vi "State Logic.vi"(0 "TLB' data in":refnum<class "TLB` - {TMPL}.lvclass">, 1 "process state logic enable":bool, 5 "trigger queue in":refnum<queue>, 7 "action queue in":refnum<queue>, 11 "error in":errorcluster) -> (4 "TLB' data out":refnum<class "TLB` - {TMPL}.lvclass">, 15 "error out":errorcluster)   [LabVIEW 2016, in "TLB` Template.lvlib" / "TLB` - {TMPL}.lvclass"]
doc: "Control process for TLB' template.\n\n<B>Input Parameters</B>\n\n<B>TLB' data in</B> is the templates' private data.\n\n<B>process state logic enable</B> enable state logic change.\n\n<B>trigger queue in</B> is a reference to a queue. Use the Create Trigger Queue function to obtain a queue reference. \n\n<B>action queue in</B> is a reference to a queue. Use the Create Action Queue function to obtain a queue reference. \n\n<B>timeout (ms)</B> queue timeout.\n\n<B>error in</B> describes error conditions that occur before this node runs. This input provides standard error in functionality.\n\n<B>Output Parameters</B>\n\n<B>TLB' data out</B> is the templates' private data.\n\n<B>error out</B> contains error information. This output provides standard error out functionality."
uses:
  TLB` - {TMPL}.lvclass
  Application Components/Trigger API/System Trigger Element.ctl
  Application Components/Trigger API/{TMPL} System Trigger.ctl
  Core Components/Actions/System Action Element.ctl
  TLB` - {TMPL}.lvclass/TLB` - {TMPL}.ctl
  State.ctl
  Core Components/Error Handler/TLB` Error Handler.lvclass/TLB` Error Handler.ctl
  Core Components/Error Handler/accessors/Get Action Causing Error.vi
  Core Components/Error Handler/accessors/Get Originating State.vi
  Core Components/Error Handler/accessors/Get Destination State.vi
  Core Components/Error Handler/accessors/Get Executed System Actions.vi
  Core Components/Error Handler/accessors/Get Remaing System Actions.vi
  Core Components/Error Handler/Core/actions/support/Error FLUSH-LOG-DIALOG.vi
  Core Components/Error Handler/Core/actions/support/Error DIALOG.vi
  Application Components/Trigger API/{TMPL} Trigger API.lvlib
  Core Components/Error Handler/TLB` Error Handler.lvclass
  Core Components/Actions/Actions.lvlib
  Core Components/Error Handler/Core/actions/support/Error FLUSH-DIALOG.vi
  TLB` Template.lvlib
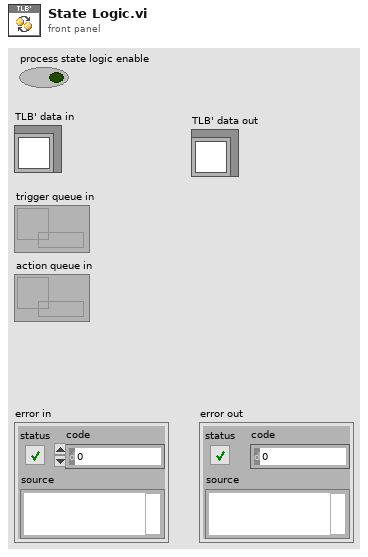
[diagram p1: front panel]
types:
  T1 = typedef "TLB` Template.lvlib/{TMPL} System Trigger.ctl" = enum16{"None", "Connect", "Start Acquisition", "Stop Acquisition", "Disconnect", "Return to Safe State Actions", "Cache User Parameters", "Close Application", "<Error>"}
  T2 = typedef "TLB` Template.lvlib/TLB` - {TMPL}.lvclass/State.ctl" = enum16{"<Startup>", "Idle", "<Shutdown>", "<Error>"}
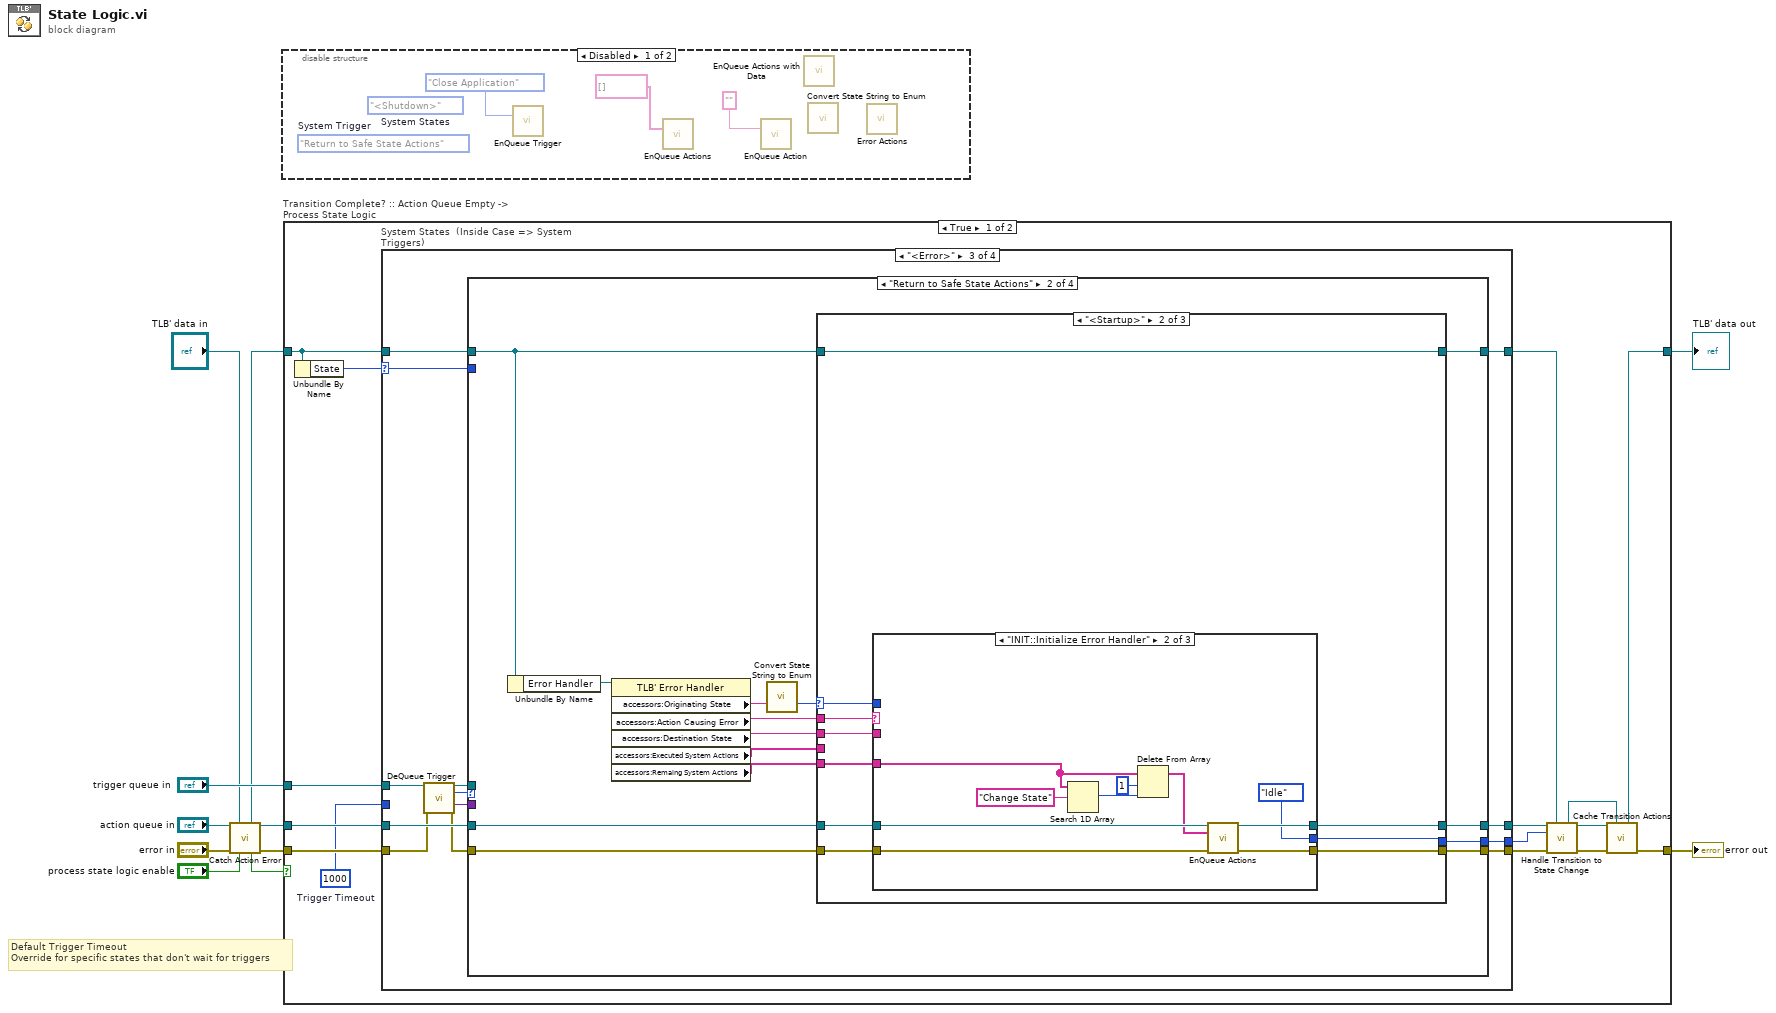
[diagram p0: block diagram]
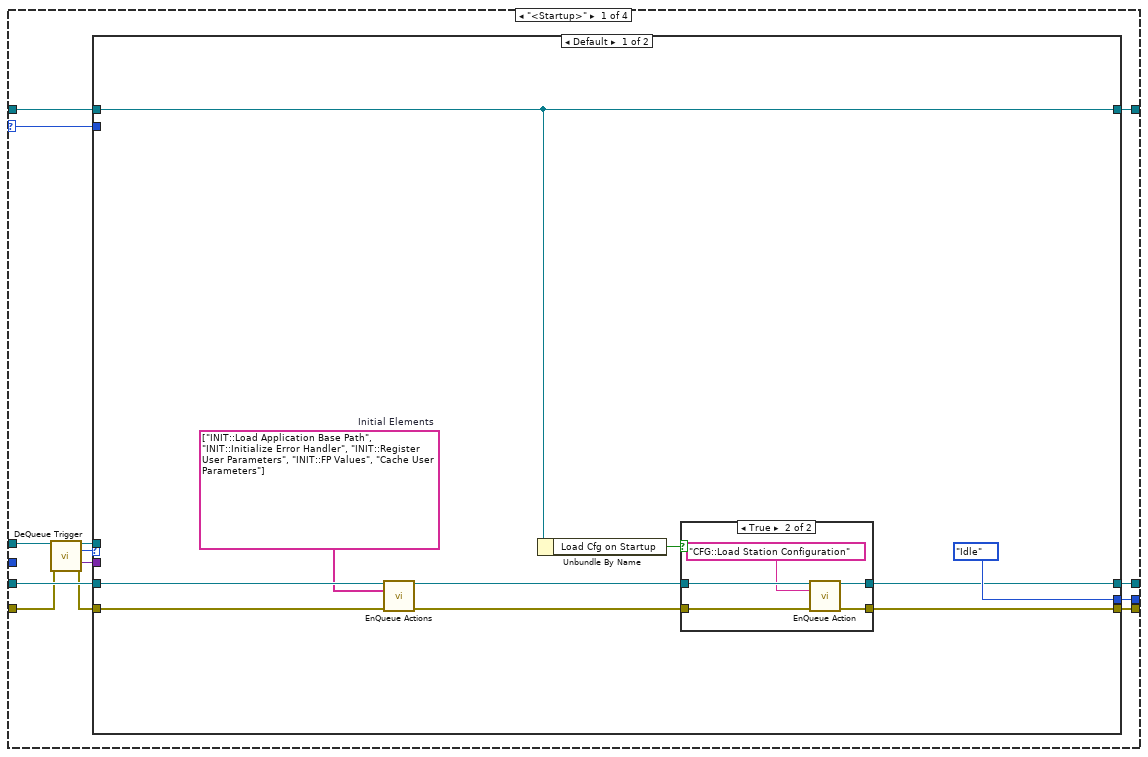
[diagram p3: hidden frame]
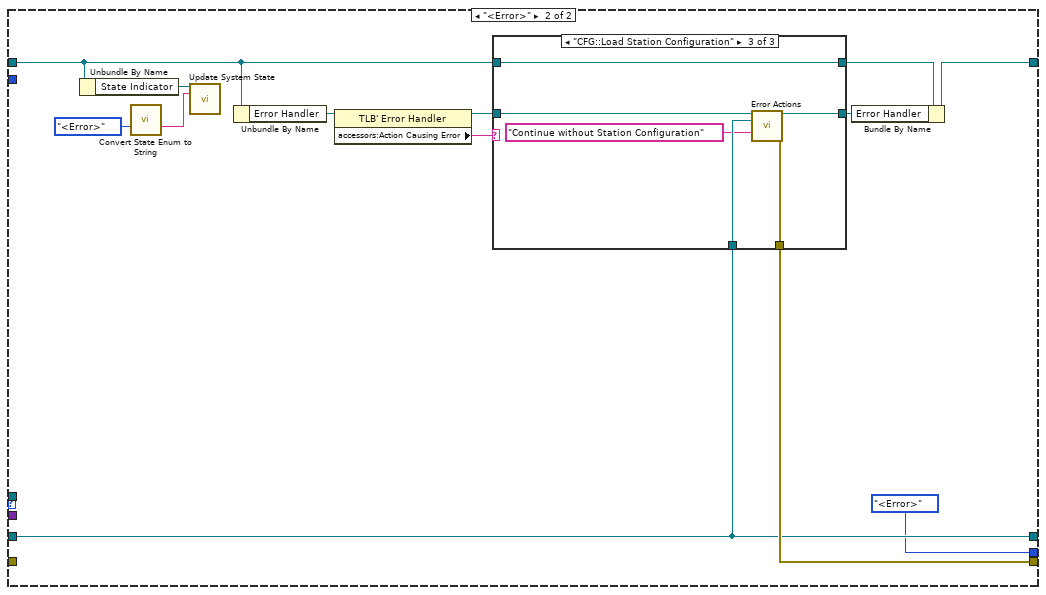
[diagram p5: hidden frame]
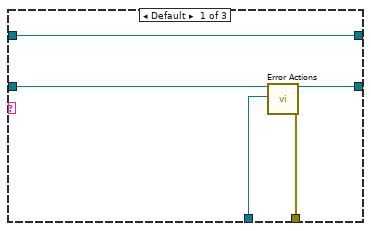
[diagram p6: hidden frame]
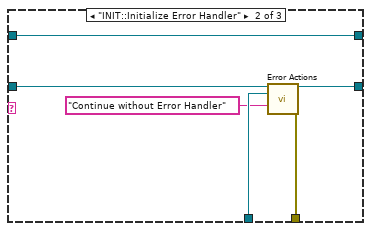
[diagram p7: hidden frame]
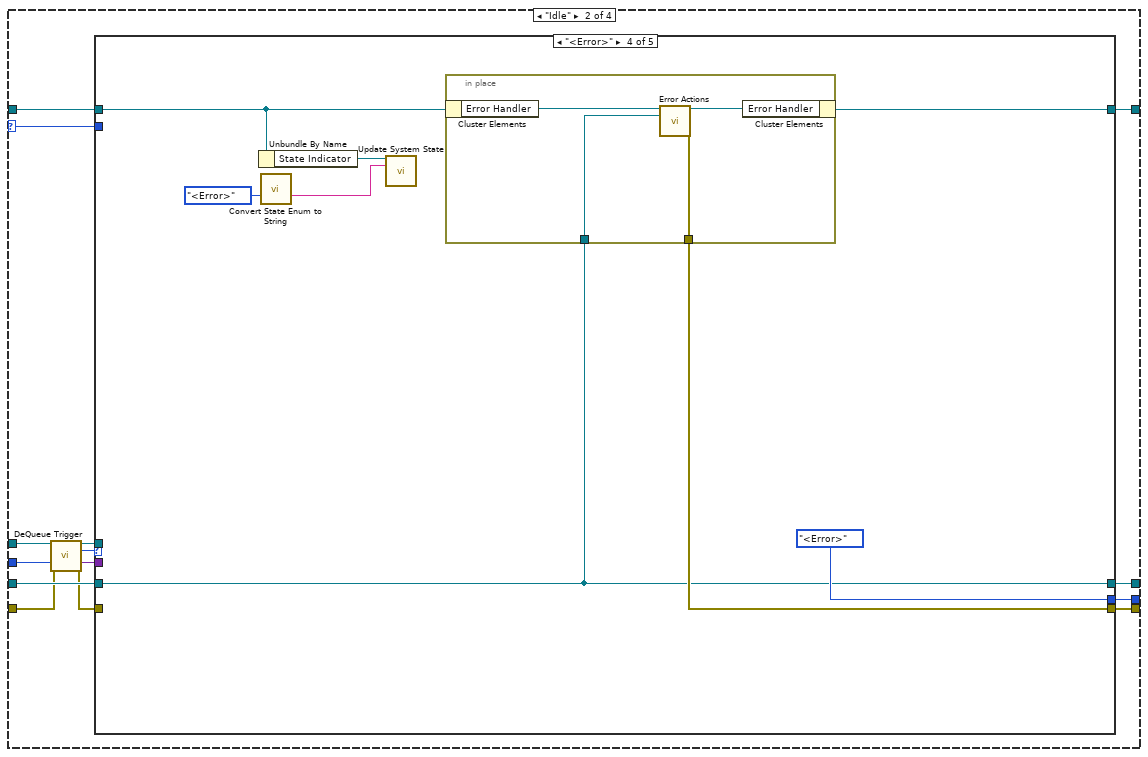
[diagram p8: hidden frame]
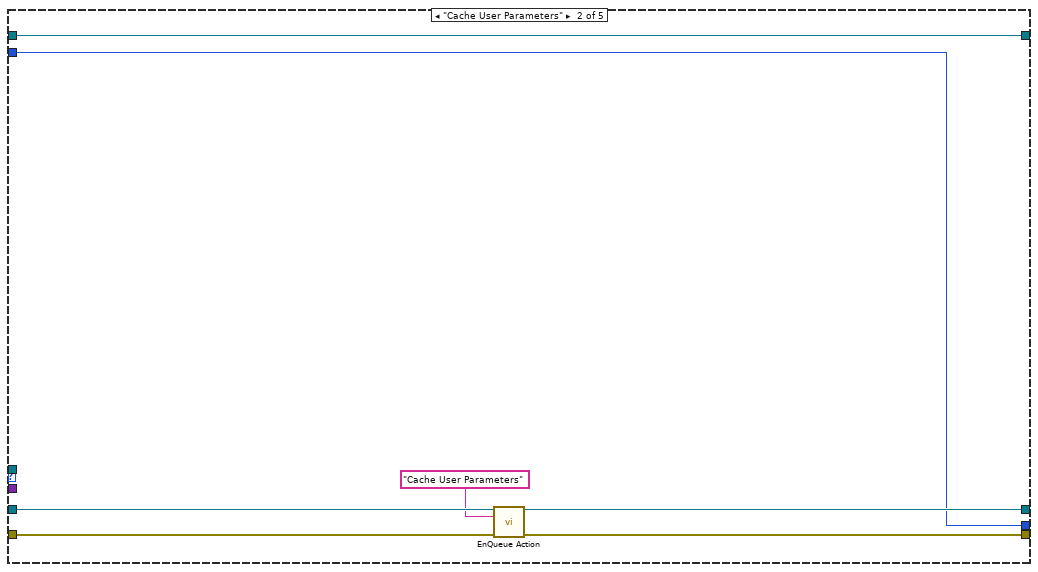
[diagram p10: hidden frame]
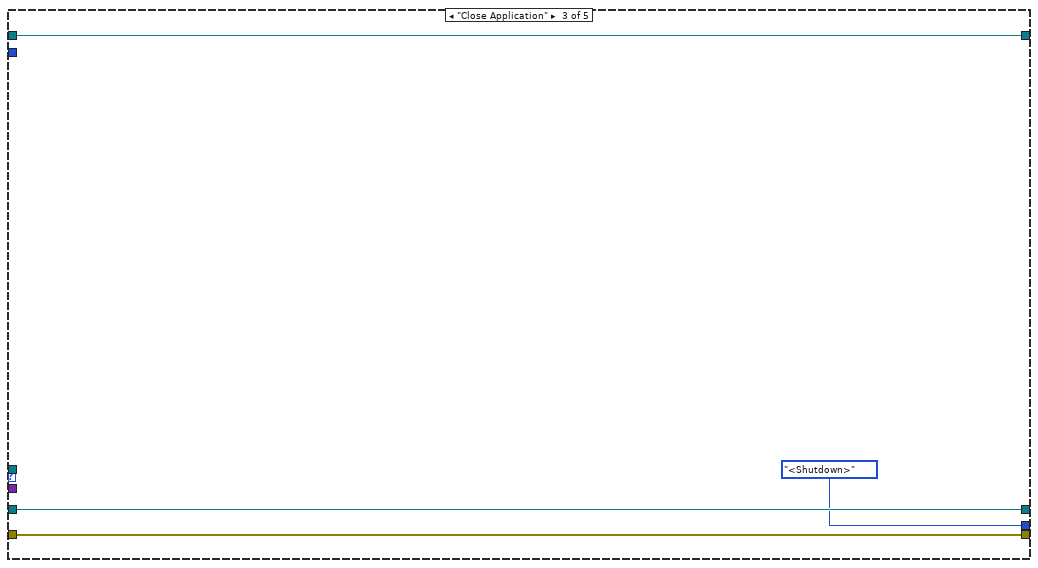
[diagram p11: hidden frame]
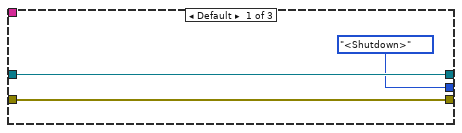
[diagram p15: hidden frame]
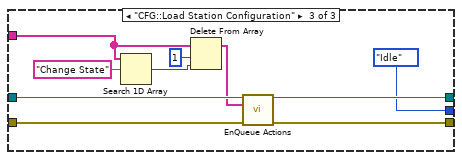
[diagram p16: hidden frame]
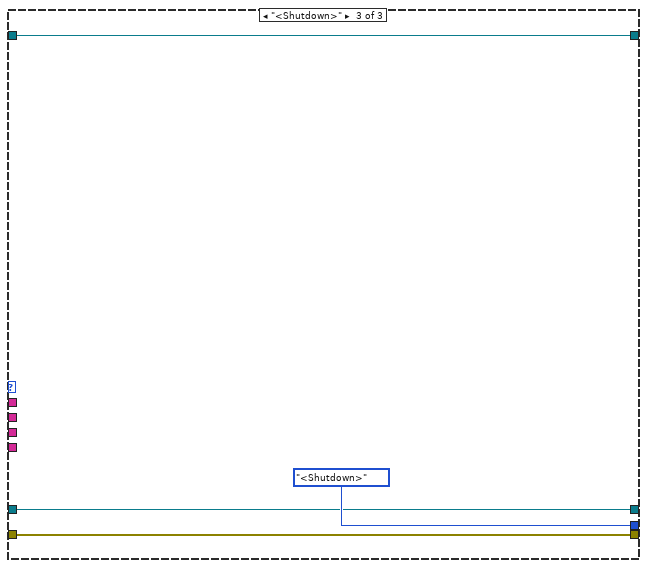
[diagram p17: hidden frame]
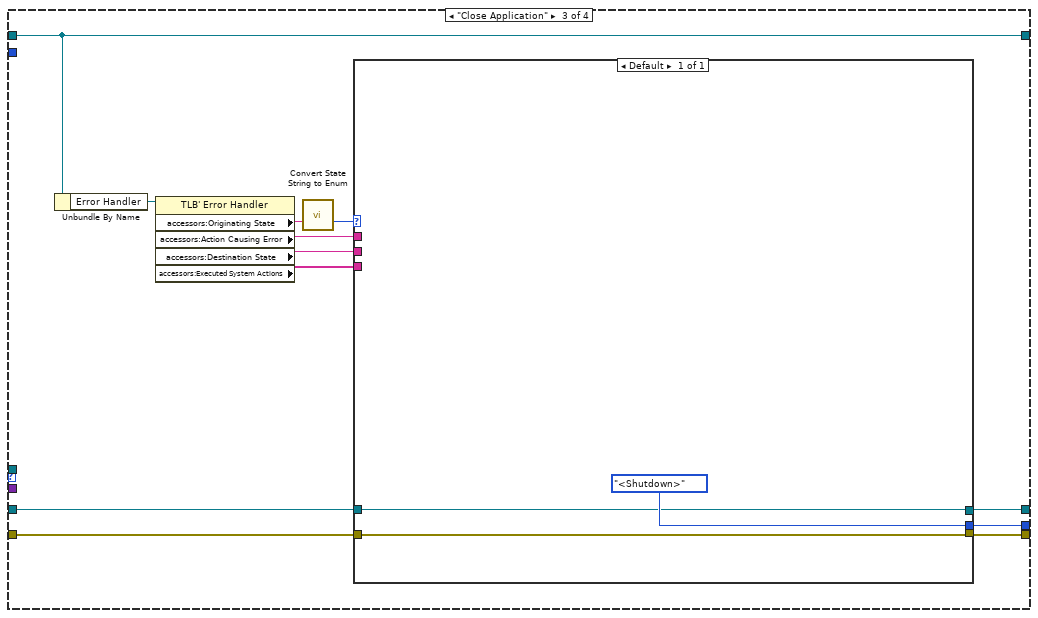
[diagram p18: hidden frame]
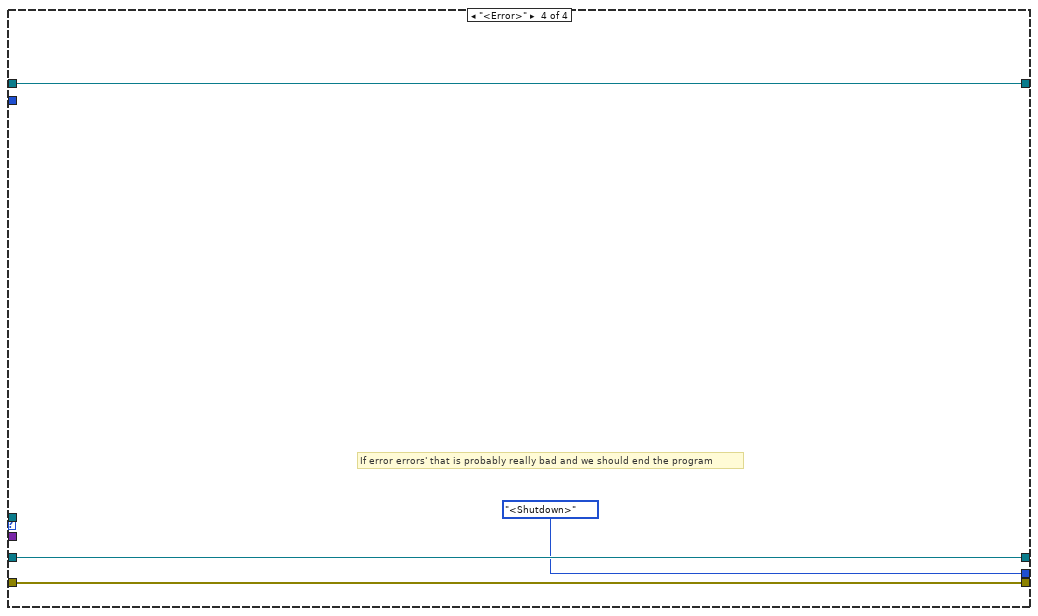
[diagram p19: hidden frame]
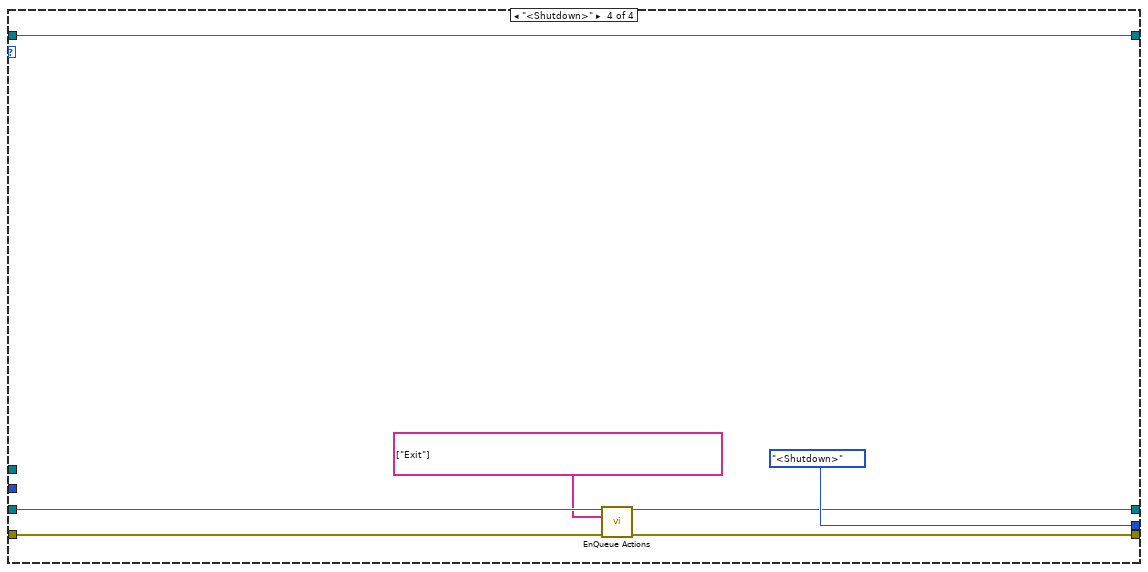
[diagram p20: hidden frame]
diagram:
  # "Default Trigger Timeout\nOverride for specific states that don't wait for triggers"
  n1 = call "Catch Action Error.vi"("action queue in"="action queue in", "TLB' Template in"="TLB' data in", "error in (no error)"="error in", "process state logic enable in"="process state logic enable") -> ("TLB' Template out"=w6:refnum<class "TLB` - {TMPL}.lvclass">, "action queue in"=w2:refnum<queue>, "process state logic enable out"=w4:bool, "error out"=w7:errorcluster)  [unwired: 8 in]
  n2 = disable-structure shown="Disabled" {
    frame Disabled {
      (unwired) {TMPL}_System_Trigger."Return to Safe State Actions"  # System Trigger
      (unwired) State."<Shutdown>"  # System States
      n3 = call "EnQueue Trigger.vi"("system trigger"={TMPL}_System_Trigger."Close Application" ("System Trigger")) -> ()  [unwired: 13 in, 2 out]
      n4 = call "EnQueue Actions.vi"("actions"=string[] [] ("message names")) -> ()  [unwired: 13 in, 2 out]
      n5 = call "EnQueue Action.vi"("action"="" ("Message Name")) -> ()  [unwired: 13 in, 2 out]
      n6 = call "EnQueue Actions with Data.vi"() -> ()  [unwired: 14 in, 2 out]
      n7 = call "Convert State String to Enum.vi"() -> ()  [unwired: 14 in, 2 out]
      n8 = call-poly "Error Actions.vi"() -> ()  [unwired: 14 in, 2 out]
    }
    frame Enabled {
    }
  }
  n9 = case "Transition Complete? :: Action Queue Empty -> Process State Logic" shown="True" w4 {
    tunnel: [w20 w233] -> w10
    tunnel: w6 -> [w25 w233]
    tunnel: w7 -> [w29 w234]
    tunnel: w2 -> [w28 _]
    tunnel: [w23 w234] -> w11
    tunnel: "trigger queue in" -> [w27 _]
    frame True {
      w21 = 1000  # Trigger Timeout
      n10 = Unbundle By Name(w25) -> ("State"=w22:T2)
      n11 = case "System States  (Inside Case => System Triggers)" shown="\"<Error>\"" w22 {
        selector: w22 -> [w30 w92 w142 _]
        tunnel: [w36 w97 w140 w231] -> w18
        tunnel: w25 -> [w37 w98 w141 w231]
        tunnel: w29 -> [w35 w96 w139 w230]
        tunnel: w28 -> [w41 w102 w143 w229]
        tunnel: [w40 w101 w146 w227] -> w26
        tunnel: w27 -> [w42 w103 w147 _]
        tunnel: [w39 w100 w145 w228] -> w19
        tunnel: [w38 w99 w144 State."<Shutdown>" ("State")] -> w15
        tunnel: w21 -> [_ w91 _ _]
        frame "<Startup>" {
          n12 = call "DeQueue Trigger.vi"("trigger queue in"=w42, "error in"=w35) -> ("trigger queue out"=w31:refnum<queue>, "system trigger"=w33:T1, "trigger data"=w32:variant, "error out"=w34:errorcluster)  [unwired: 10 in]
          n13 = case shown="Default" w33 {
            tunnel: w34 -> [w49 _]
            tunnel: w41 -> [w51 w70]
            tunnel: [w46 w71] -> w40
            tunnel: [w44 w70] -> w39
            tunnel: w32 -> [_ _]
            tunnel: [State."Idle" ("State") State."<Error>" ("State")] -> w38
            tunnel: w37 -> [w47 w61]
            tunnel: [w47 w72] -> w36
            tunnel: w31 -> [_ _]
            tunnel: w30 -> [_ _]
            frame Default {
              w50 = string[] ["INIT::Load Application Base Path", "INIT::Initialize Error Handler", "INIT::Register User Parameters", "INIT::FP Values", "Cache User Parameters"]  # Initial Elements
              n14 = call "EnQueue Actions.vi"("action queue in"=w51, "actions"=w50, "error in"=w49) -> ("action queue out"=w45:refnum<queue>, "error out"=w48:errorcluster)  [unwired: 11 in]
              n15 = Unbundle By Name(w47) -> ("Load Cfg on Startup"=w43:bool)
              n16 = case shown="True" w43 {
                tunnel: w48 -> [w53 w59]
                tunnel: [w53 w58] -> w46
                tunnel: w45 -> [w54 w57]
                tunnel: [w54 w56] -> w44
                frame False {
                }
                frame True {
                  n17 = call "EnQueue Action.vi"("action queue in"=w57, "action"="CFG::Load Station Configuration", "error in"=w59) -> ("action queue out"=w56:refnum<queue>, "error out"=w58:errorcluster)  [unwired: 11 in]
                }
              }
            }
            frame "<Error>" {
              n18 = Unbundle By Name(w61) -> ("State Indicator"=w65:refnum<user-event>)
              n19 = call "Convert State Enum to String.vi"("state in"=State."<Error>") -> ("state out"=w64:string)  [unwired: 13 in, 1 out]
              n20 = call "Update System State.vi"("State Indicator"=w65, "system state message"=w64) -> ()  [unwired: 13 in, 1 out]
              n21 = Unbundle By Name(w61) -> ("Error Handler"=w67:refnum<class "TLB` Error Handler.lvclass">)
              n22 = property class="TLB' Error Handler"(reference=w67) -> (reference out=w66:refnum<class "TLB` Error Handler.lvclass">, "accessors:Action Causing Error"=w63:string)  [unwired: 1 in, 1 out]
              n23 = case shown="\"CFG::Load Station Configuration\"" w63 {
                tunnel: [w75 w83 w89] -> w71
                tunnel: w70 -> [w74 w82 w88]
                tunnel: [w76 w81 w87] -> w68
                tunnel: w66 -> [w77 w80 w86]
                tunnel: w61 -> [w73 w78 w84]
                tunnel: [w73 w78 w84] -> w60
                frame Default {
                  n24 = call-poly "Error Actions.vi"("Error Handler in"=w77, "action queue in"=w74) -> ("Error Handler out"=w76:refnum<class "TLB` Error Handler.lvclass">, "error out"=w75:errorcluster)  [unwired: 12 in]
                }
                frame "INIT::Initialize Error Handler" {
                  n25 = call-poly "Error Actions.vi"("Error Handler in"=w80, "action queue in"=w82, "error button text (Return to Safe State)"="Continue without Error Handler") -> ("Error Handler out"=w81:refnum<class "TLB` Error Handler.lvclass">, "error out"=w83:errorcluster)  [unwired: 11 in]
                }
                frame "CFG::Load Station Configuration" {
                  n26 = call-poly "Error Actions.vi"("Error Handler in"=w86, "action queue in"=w88, "error button text (Return to Safe State)"="Continue without Station Configuration") -> ("Error Handler out"=w87:refnum<class "TLB` Error Handler.lvclass">, "error out"=w89:errorcluster)  [unwired: 11 in]
                }
              }
              n27 = Bundle By Name(cluster=w60, "Error Handler"=w68) -> (w72:refnum<class "TLB` - {TMPL}.lvclass">)
            }
          }
        }
        frame "Idle" {
          n28 = call "DeQueue Trigger.vi"("trigger queue in"=w103, "timeout, ms (0)"=w91, "error in"=w96) -> ("trigger queue out"=w90:refnum<queue>, "system trigger"=w94:T1, "trigger data"=w93:variant, "error out"=w95:errorcluster)  [unwired: 9 in]
          n29 = case shown="\"<Error>\"" w94 {
            tunnel: w95 -> [w106 w114 w117 _ w133]
            tunnel: w102 -> [w107 w111 w118 w122 w134]
            tunnel: [w106 w112 w117 w124 w133] -> w101
            tunnel: [w107 w110 w118 w122 w134] -> w100
            tunnel: w93 -> [_ _ _ _ _]
            tunnel: w98 -> [w105 w113 w116 w121 w132]
            tunnel: [w104 w108 State."<Shutdown>" ("State") State."<Error>" ("State") w131] -> w99
            tunnel: [w105 w113 w116 w123 w132] -> w97
            tunnel: w92 -> [w104 w108 _ _ w131]
            tunnel: w90 -> [_ _ _ _ _]
            frame "None" {
            }
            frame "Cache User Parameters" {
              n30 = call "EnQueue Action.vi"("action queue in"=w111, "action"="Cache User Parameters", "error in"=w114) -> ("action queue out"=w110:refnum<queue>, "error out"=w112:errorcluster)  [unwired: 11 in]
            }
            frame "Close Application" {
            }
            frame "<Error>" {
              n31 = Unbundle By Name(w121) -> ("State Indicator"=w125:refnum<user-event>)
              n32 = call "Convert State Enum to String.vi"("state in"=State."<Error>") -> ("state out"=w119:string)  [unwired: 13 in, 1 out]
              n33 = call "Update System State.vi"("State Indicator"=w125, "system state message"=w119) -> ()  [unwired: 13 in, 1 out]
              n34 = in-place {
                in-place-border: [w128] -> w124
                in-place-border: w122 -> [w127]
                n35 = in-place-cluster #1(w121) -> ("Error Handler"=w130:refnum<class "TLB` Error Handler.lvclass">)
                n36 = call-poly "Error Actions.vi"("Error Handler in"=w130, "action queue in"=w127) -> ("Error Handler out"=w129:refnum<class "TLB` Error Handler.lvclass">, "error out"=w128:errorcluster)  [unwired: 12 in]
                n37 = in-place-cluster #1("Error Handler"=w129) -> (w123:refnum<class "TLB` - {TMPL}.lvclass">)
              }
            }
            frame Default {
            }
          }
        }
        frame "<Error>" {
          n38 = call "DeQueue Trigger.vi"("trigger queue in"=w147, "error in"=w139) -> ("trigger queue out"=w138:refnum<queue>, "system trigger"=w137:T1, "trigger data"=w135:variant, "error out"=w136:errorcluster)  [unwired: 10 in]
          n39 = case shown="\"Return to Safe State Actions\"" w137 {
            tunnel: w141 -> [w149 w152 w207 w223]
            tunnel: [w150 w162 w216 w222] -> w146
            tunnel: w136 -> [w150 w164 w217 w222]
            tunnel: w143 -> [w151 w165 w218 w225]
            tunnel: [w151 w163 w213 w225] -> w145
            tunnel: [w148 w161 w215 State."<Shutdown>" ("State")] -> w144
            tunnel: w138 -> [_ _ _ _]
            tunnel: w142 -> [w148 _ _ _]
            tunnel: w135 -> [_ _ _ _]
            tunnel: [w149 w160 w207 w223] -> w140
            frame Default {
            }
            frame "Return to Safe State Actions" {
              n40 = Unbundle By Name(w152) -> ("Error Handler"=w159:refnum<class "TLB` Error Handler.lvclass">)
              n41 = property class="TLB' Error Handler"(reference=w159) -> ("accessors:Originating State"=w154:string, "accessors:Action Causing Error"=w158:string, "accessors:Destination State"=w157:string, "accessors:Executed System Actions"=w156:string[], "accessors:Remaing System Actions"=w153:string[])  [unwired: 1 in, 2 out]
              n42 = call "Convert State String to Enum.vi"("state in"=w154) -> ("state out"=w155:T2)  [unwired: 13 in, 1 out]
              n43 = case shown="\"<Startup>\"" w155 {
                selector: w155 -> [w166 w171 _]
                tunnel: w165 -> [w169 w177 w204]
                tunnel: w164 -> [w167 w178 w203]
                tunnel: [w167 w176 w203] -> w162
                tunnel: [w169 w175 w204] -> w163
                tunnel: [w166 w174 State."<Shutdown>" ("State")] -> w161
                tunnel: w152 -> [w168 w179 w206]
                tunnel: [w168 w179 w206] -> w160
                tunnel: w158 -> [_ w173 _]
                tunnel: w157 -> [_ w170 _]
                tunnel: w156 -> [_ _ _]
                tunnel: w153 -> [_ w172 _]
                frame Default {
                }
                frame "<Startup>" {
                  n44 = case shown="\"INIT::Initialize Error Handler\"" w173 {
                    tunnel: w178 -> [w181 w191 w201]
                    tunnel: w177 -> [w182 w192 w202]
                    tunnel: [w181 w190 w200] -> w176
                    tunnel: [w182 w189 w199] -> w175
                    tunnel: [State."<Shutdown>" ("State") State."Idle" ("state out") State."Idle" ("state out")] -> w174
                    tunnel: w172 -> [_ w188 w198]
                    tunnel: w171 -> [_ _ _]
                    tunnel: w170 -> [_ _ _]
                    frame Default {
                    }
                    frame "INIT::Initialize Error Handler" {
                      n45 = Search 1D Array(1D array=w188, element="Change State") -> (index of element=w186:i32)  [unwired: 1 in]
                      n46 = Delete From Array(array=w188, length=1, index=w186) -> (array with subset deleted=w187:string[])  [unwired: 1 out]
                      n47 = call "EnQueue Actions.vi"("action queue in"=w192, "actions"=w187, "error in"=w191) -> ("action queue out"=w189:refnum<queue>, "error out"=w190:errorcluster)  [unwired: 11 in]
                    }
                    frame "CFG::Load Station Configuration" {
                      n48 = Search 1D Array(1D array=w198, element="Change State") -> (index of element=w196:i32)  [unwired: 1 in]
                      n49 = Delete From Array(array=w198, length=1, index=w196) -> (array with subset deleted=w197:string[])  [unwired: 1 out]
                      n50 = call "EnQueue Actions.vi"("action queue in"=w202, "actions"=w197, "error in"=w201) -> ("action queue out"=w199:refnum<queue>, "error out"=w200:errorcluster)  [unwired: 11 in]
                    }
                  }
                }
                frame "<Shutdown>" {
                }
              }
            }
            frame "Close Application" {
              n51 = Unbundle By Name(w207) -> ("Error Handler"=w214:refnum<class "TLB` Error Handler.lvclass">)
              n52 = property class="TLB' Error Handler"(reference=w214) -> ("accessors:Originating State"=w212:string, "accessors:Action Causing Error"=w208:string, "accessors:Destination State"=w209:string, "accessors:Executed System Actions"=w210:string[])  [unwired: 1 in, 2 out]
              n53 = call "Convert State String to Enum.vi"("state in"=w212) -> ("state out"=w211:T2)  [unwired: 13 in, 1 out]
              n54 = case shown="Default" w211 {
                tunnel: w218 -> [w220]
                tunnel: w217 -> [w219]
                tunnel: [w219] -> w216
                tunnel: [w220] -> w213
                tunnel: [State."<Shutdown>" ("State")] -> w215
                tunnel: w208 -> [_]
                tunnel: w209 -> [_]
                tunnel: w210 -> [_]
                frame Default {
                }
              }
            }
            frame "<Error>" {
              # "If error errors' that is probably really bad and we should end the program"
            }
          }
        }
        frame "<Shutdown>" {
          n55 = call "EnQueue Actions.vi"("action queue in"=w229, "actions"=string[] ["Exit"], "error in"=w230) -> ("action queue out"=w228:refnum<queue>, "error out"=w227:errorcluster)  [unwired: 11 in]
        }
      }
      n56 = call "Handle Transition to State Change.vi"("action queue in"=w19, "TLB' Template in"=w18, "Destination State"=w15, "error in (no error)"=w26) -> ("TLB' Template out"=w17:refnum<class "TLB` - {TMPL}.lvclass">, "action queue in"=w16:refnum<queue>, "error out"=w24:errorcluster)  [unwired: 9 in]
      n57 = call "Cache Transition Actions.vi"("action queue in"=w16, "TLB' Template in"=w17, "error in (no error)"=w24) -> ("TLB' Template out"=w20:refnum<class "TLB` - {TMPL}.lvclass">, "error out"=w23:errorcluster)  [unwired: 11 in]
    }
    frame False {
    }
  }
  "error out" <- w11
  "TLB' data out" <- w10
